vi "Ex11_Sub.vi"(10 "Stop Time":dbl, 11 "Digital 입력":refnum<vi>) -> (1 "Elapsed Time (s)":dbl caption="경과 시간(초)", 2 "Time has Elapsed":bool, 3 "웨이브폼 차트":dbl(graph))   [LabVIEW 2016]
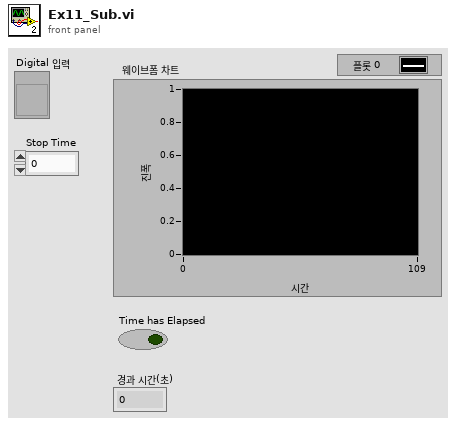
[diagram p1: front panel]
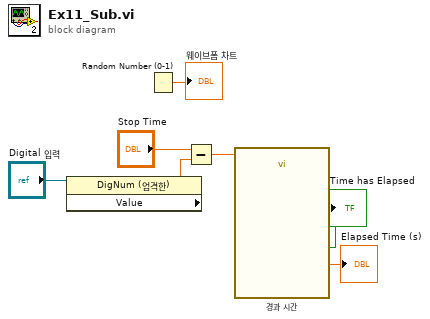
[diagram p0: block diagram]
diagram:
  n1 = property class="DigNum (엄격한)"(reference="Digital 입력") -> ("Value"=w5:dbl)  [unwired: 1 in, 2 out]
  n2 = Random Number (0-1)() -> (number: 0 to 1=→"웨이브폼 차트":dbl)
  n3 = Subtract(x="Stop Time", y=w5) -> (x-y=w4:dbl)
  n4 = call "경과 시간"("Time Target (s)"=w4) -> ("Elapsed Time (s)"=→"Elapsed Time (s)":dbl, "Time has Elapsed"=→"Time has Elapsed":bool)  [unwired: 11 in, 6 out]
